vi "PowerX 2D.vi"(8 "Multiplier":dbl=100.0, 9 "Divider":dbl=100.0, 10 "Power":dbl, 11 "Signal In":dbl[][](array[numeric])) -> (3 "Signal Out":dbl[][](array[numeric]))   [LabVIEW 2023]
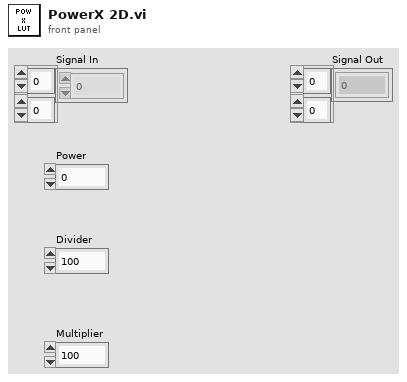
[diagram p1: front panel]
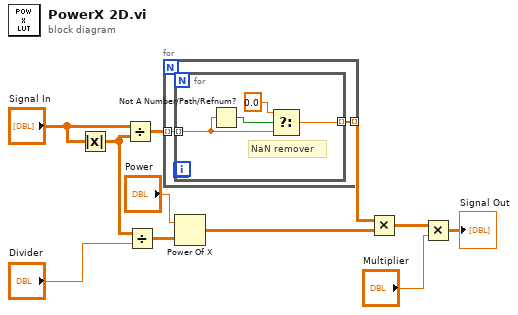
[diagram p0: block diagram]
diagram:
  n1 = Absolute Value(x="Signal In") -> (abs(x)=w1:dbl[][])
  n2 = Divide(x="Signal In", y=w1) -> (x/y=w3:dbl[][])
  n3 = Divide(x=w1, y="Divider") -> (x/y=w5:dbl[][])
  n4 = for {
    tunnel: [w13] -> w4 mode=indexing
    tunnel: w3 -> [w12] mode=indexing
    n5 = for {
      tunnel: w12 -> [w15] mode=indexing
      tunnel: [w16] -> w13 mode=indexing
      # "NaN remover"
      n6 = Not A Number/Path/Refnum?(number/path/refnum=w15) -> (NaN/Path/Refnum?=w14:bool)
      n7 = Select(t=0.0, s=w14, f=w15) -> (s? t:f=w16:dbl)
    }
  }
  n8 = Power Of X(1:w5, 2:"Power") -> (0:w6:dbl[][])
  n9 = Multiply(x=w4, y=w6) -> (x*y=w2:dbl[][])
  n10 = Multiply(x=w2, y="Multiplier") -> (x*y=→"Signal Out":dbl[][])
